vi "Read one frame from each bin file.vi"(7 "Funct data structure":bool, 8 "error in (no error)":errorcluster, 9 "Master video's frame number (unity-based)":i32, 11 "Get/set":T1) -> (0 "Error out":errorcluster, 3 "Cam videos cluster":T2 {"Vid4 Rel time (ms)" format="%.0f ms"; "Vid3 Rel time (ms)" format="%.0f ms"; "Vid2 Rel time (ms)" format="%.0f ms"; "Vid1 Rel time (ms)" format="%.0f ms"})   [LabVIEW 2013]
uses:
  Typedefs/Cam videos cluster.ctl
  Functional Imaging Viewer/Typedefs/Get-Set-Clear Control.ctl
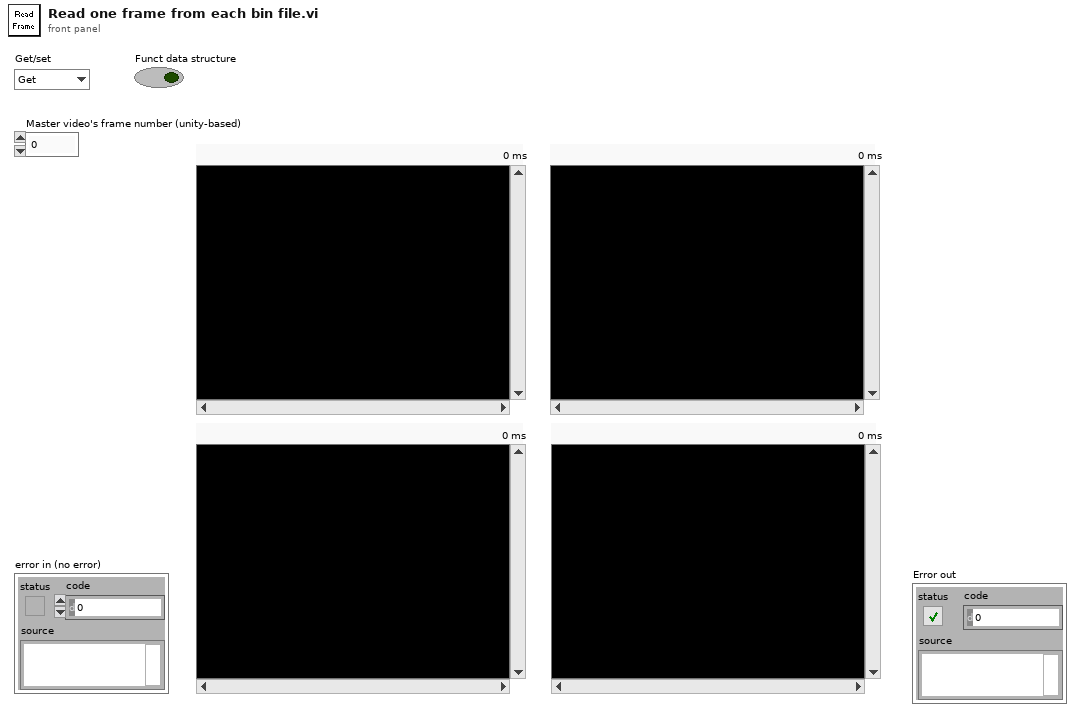
[diagram p1: front panel]
types:
  T1 = typedef "Get-Set-Clear Control.ctl" = enum16{"Get", "Set", "Clear"}
  T2 = typedef "Cam videos cluster.ctl" = cluster{"Vid 1":T3, "Vid 2":T3, "Vid 3":T3, "Vid 4":T3, "Vid1 Rel time (ms)":u32, "Vid2 Rel time (ms)":u32, "Vid3 Rel time (ms)":u32, "Vid4 Rel time (ms)":u32}
  T3 = typedef "IMAQ Image.ctl" = refnum<image>
  T4 = enum16{"None", "Release queue", "Obtain queue", "Enqueue", "Get status", "Set status"}
  T5 = typedef "Number of frames and locations cluster.ctl" = cluster{"Original number of frames":i32, "Number of valid frames":i32, "Frame number":i64[], "Frame location":i64[], "Frame rel.time":i64[]}
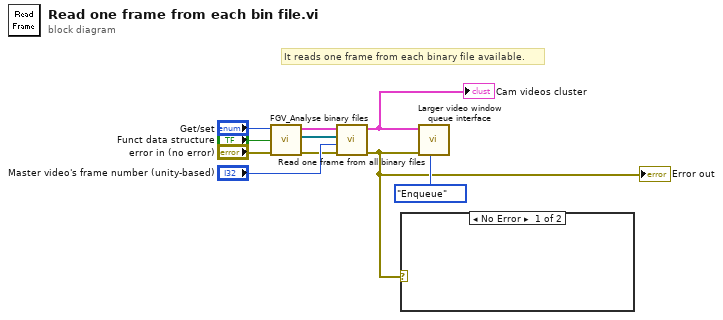
[diagram p0: block diagram]
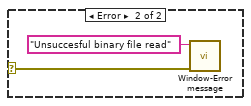
[diagram p2: hidden frame]
diagram:
  # "It reads one frame from each binary file available."
  n1 = call "FGV_Analyse binary files.vi"("error in (no error)"="error in (no error)", "Funct data structure"="Funct data structure", "Get/Set info & refs"="Get/set") -> ("Error out"=w5:errorcluster, "Cam Binary Videos Refs"=w7:refnum<file>[], "Frame numbers & locations in each video file"=w8:T5[])  [unwired: 5 in, 1 out]
  n2 = call "Read one frame from all binary files.vi"("error in (no error)"=w5, "Master video's frame number (unity-based)"="Master video's frame number (unity-based)", "Cam Binary Videos (ref)"=w7, "Frame numbers & locations in each video file"=w8) -> ("Error out"=w2:errorcluster, "Cam videos cluster"=w4:T2)  [unwired: 5 in, 1 out]
  "Cam videos cluster" <- w4
  "Error out" <- w2
  n3 = case shown="No Error" w2 {
    selector: w2 -> [_ w12]
    frame No Error {
    }
    frame Error {
      n4 = call "Window-Error message.vi"("error in (no error)"=w12, "Message"="Unsuccesful binary file read") -> ()  [unwired: 9 in, 1 out]
    }
  }
  n5 = call "Larger video window queue interface.vi"("Function"=T4."Enqueue", "error in (no error)"=w2, "Cam videos cluster in"=w4) -> ()  [unwired: 8 in, 1 out]
